vi "CH375_Abs.vi"(8 "Error In":errorcluster caption="错误输入", 11 "旋转角度":dbl) -> (0 "Error Out":errorcluster caption="错误输出")   [LabVIEW 2020]
uses:
  Global_CH375.vi
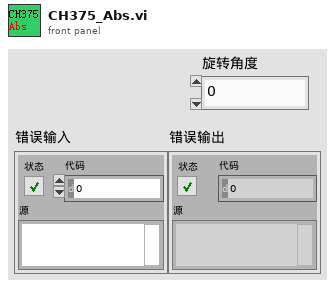
[diagram p1: front panel]
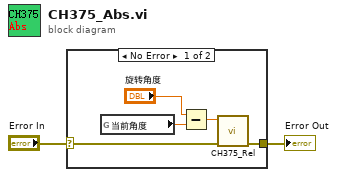
[diagram p0: block diagram]
diagram:
  n1 = case shown="No Error" "Error In" {
    selector: "Error In" -> [w6 w8]
    tunnel: [w5 w8] -> w1
    frame No Error {
      n2 = global read "Global_CH375.vi" "当前角度"() -> (w4:dbl)
      n3 = Subtract(x="旋转角度", y=w4) -> (x-y=w7:dbl)
      n4 = call "CH375_Rel.vi"("Error In"=w6, "移动步长"=w7) -> ("Error Out"=w5:errorcluster)  [unwired: 9 in]
    }
    frame Error {
    }
  }
  "Error Out" <- w1
